vi "Test - CSG array over string conversion.vi"() -> ()   [LabVIEW 2019, in "mmW_commands.lvlib"]
uses:
  mmW_commands.lvlib
panel:
  out "return value":i32
  out "error out":errorcluster
  out "string1 2":string
  out "length string1 2":i32
  out "value 2":csg[](array[numeric])
  out "length string2 2":i32
  out "variant 2":variant
  in  "module path":path=path "C:/Barkhausen mmWave radar/Development/mmWave_driver_Py/LV-API/mmW_commands/utils/append_JSON.py"
  out "variant":variant
  out "length string2":i32
  out "value":csg[](array[numeric])
  out "length string1":i32
  out "string1":string
  in  "Waveform in":csg[](array[numeric])=[-50.0+50.0i, 0.0-1.0i, -1.0+2.0i]
  # "C:\\Barkhausen mmWave radar\\Development\\mmWave_driver_Py\\LV-API\\mmW_commands\\utils\\append_JSON.py"
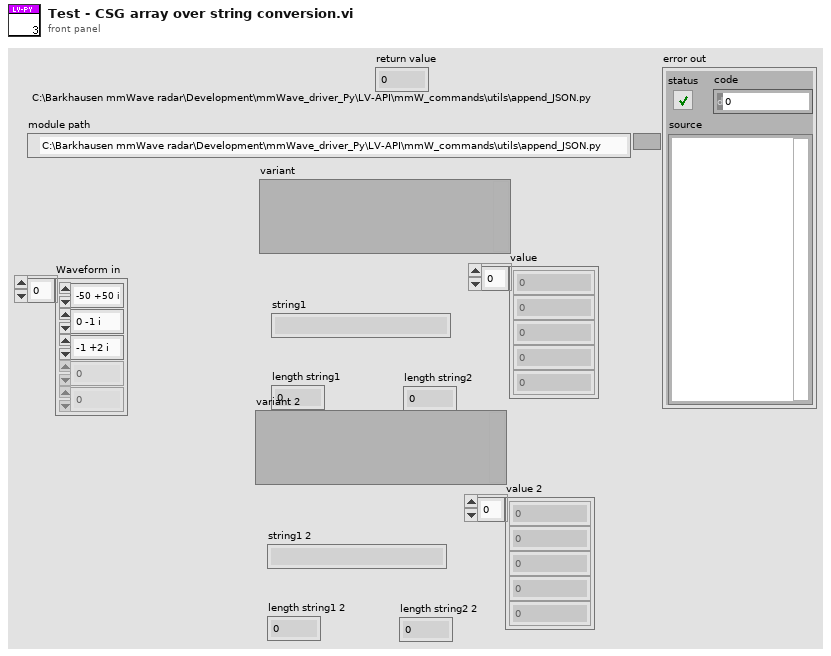
[diagram p1: front panel]
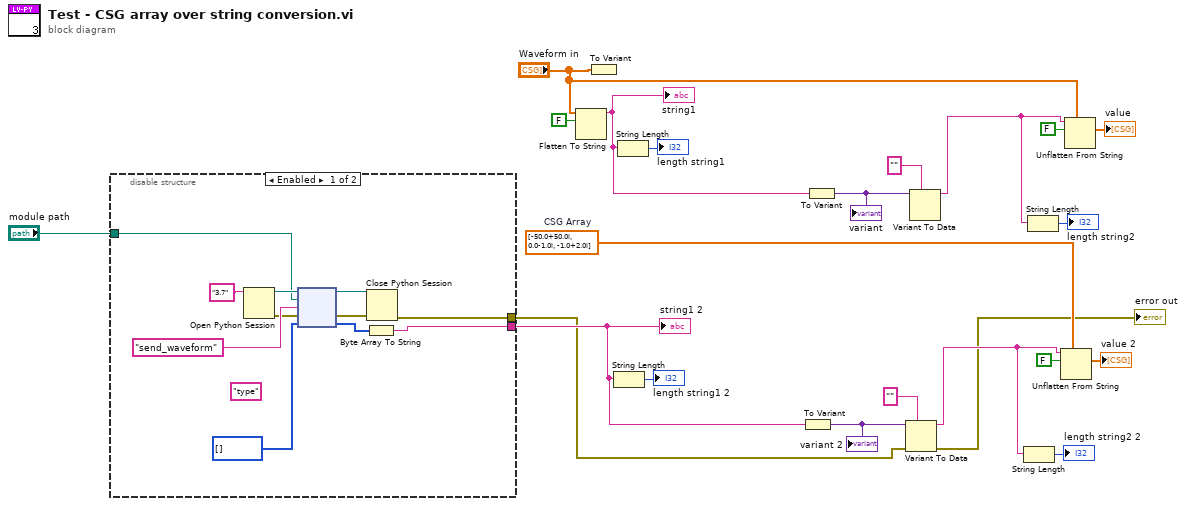
[diagram p0: block diagram]
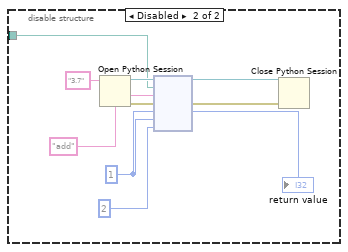
[diagram p2: hidden frame]
diagram:
  w4 = csg[] [-50.0+50.0i, 0.0-1.0i, -1.0+2.0i]  # CSG Array
  n1 = disable-structure shown="Enabled" {
    disable-tunnel: "module path" -> [w30 w38]
    disable-tunnel: [w26 _] -> w3
    disable-tunnel: [w23 _] -> w2
    frame Enabled {
      (unwired) "type" ("function name")
      n2 = Open Python Session(python version="3.7" ("Python version")) -> (session out=w32:refnum<k35>, error out=w25:errorcluster)  [unwired: 2 in]
      n3 = node(w32, w30, "send_waveform" ("function name"), w25, u8[] []) -> (w31:refnum<k35>, w24:errorcluster, w27:u8[])  [unwired: 2 out]
      n4 = Byte Array To String(unsigned byte array=w27) -> (string=w26:string)
      n5 = Close Python Session(session in=w31, error in=w24) -> (11:w23:errorcluster)
    }
    frame Disabled {
      w36 = 1
      n6 = Open Python Session(python version="3.7" ("Python version")) -> (session out=w43:refnum<k35>, error out=w41:errorcluster)  [unwired: 2 in]
      n7 = node(w43, w38, "add" ("function name"), w41, w36, w36, 2) -> (w42:refnum<k35>, w40:errorcluster, →"return value":i32)  [unwired: 2 in, 2 out]
      n8 = Close Python Session(session in=w42, error in=w40) -> ()  [unwired: 1 out]
    }
  }
  "string1 2" <- w3
  n9 = Flatten To String(anything="Waveform in", prepend array or string size? (T)=FALSE) -> (data string=w19:string)  [unwired: 2 in, 2 out]
  "string1" <- w19
  n10 = To Variant(anything="Waveform in") -> ()  [unwired: 1 out]
  n11 = String Length(string=w3) -> (length=→"length string1 2":i32)
  n12 = String Length(string=w19) -> (length=→"length string1":i32)
  n13 = To Variant(anything=w3) -> (Variant=w7:variant)
  "variant 2" <- w7
  n14 = To Variant(anything=w19) -> (Variant=w18:variant)
  "variant" <- w18
  n15 = Variant To Data(error in=w2, type="", Variant=w7) -> (data=w10:string, error out=→"error out":errorcluster)
  n16 = Variant To Data(type="", Variant=w18) -> (data=w15:string)  [unwired: 1 in, 1 out]
  n17 = String Length(string=w10) -> (length=→"length string2 2":i32)
  n18 = String Length(string=w15) -> (length=→"length string2":i32)
  n19 = Unflatten From String(type=w4, binary string=w10, data includes array or string size? (T)=FALSE) -> (value=→"value 2":csg[])  [unwired: 2 in, 2 out]
  n20 = Unflatten From String(type="Waveform in", binary string=w15, data includes array or string size? (T)=FALSE) -> (value=→"value":csg[])  [unwired: 2 in, 2 out]
